vi "Mysql data reader Scalar double.vi"(8 "error in (no error)":errorcluster, 11 ".NET Refnum in":refnum<k24>) -> (0 "error out":errorcluster, 3 "GetString":dbl)   [LabVIEW 2020, in "mysql.lvlib" / "mysql.lvclass"]
uses:
  mysql.lvclass
  MySql.Data
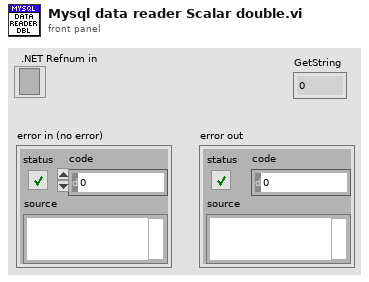
[diagram p1: front panel]
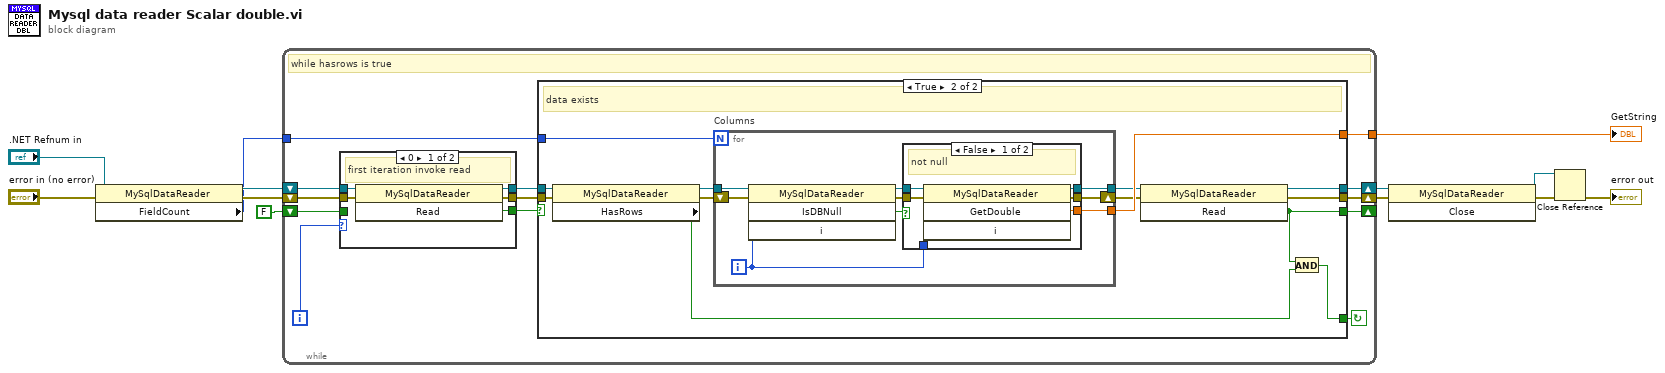
[diagram p0: block diagram]
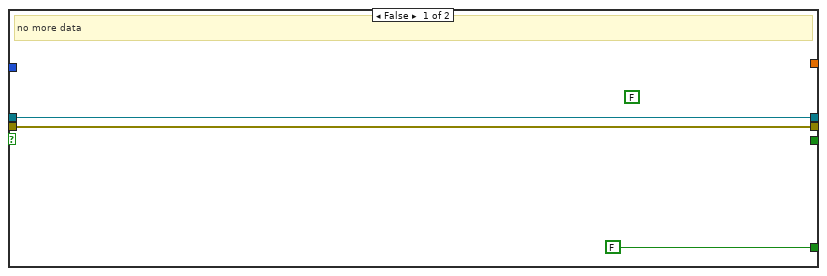
[diagram p3: hidden frame]
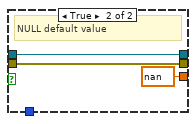
[diagram p4: hidden frame]
diagram:
  n1 = property class="MySqlDataReader"(reference=".NET Refnum in", error in="error in (no error)") -> (reference out=w8:refnum<k24>, error out=w7:errorcluster, "FieldCount"=w4:i32)
  n2 = while {
    tunnel: w4 -> [w25]
    tunnel: [w24] -> w5
    shift-right: [w22] -> w10
    shift-left: w7 -> [w20]
    shift-right: [w23] -> w9
    shift-left: w8 -> [w19]
    shift-right: [w13] -> _
    shift-left: FALSE -> [w15]
    i -> [w14]
    stop <- w21 continue-if-true
    # "while hasrows is true"
    n3 = case shown="0" w14 {
      tunnel: w20 -> [w30 w32]
      tunnel: [w29 w32] -> w17
      tunnel: w19 -> [w28 w33]
      tunnel: [w27 w33] -> w18
      tunnel: [w26 w31] -> w16
      tunnel: w15 -> [_ w31]
      frame 0 {
        # "first iteration invoke read"
        n4 = invoke class="MySqlDataReader" method="Read"(reference=w28, error in=w30) -> (reference out=w27:refnum<k24>, error out=w29:errorcluster, "Read"=w26:bool)  [unwired: 1 in]
      }
      frame 1.., Default {
        # "read after for other iterations"
      }
    }
    n5 = case shown="True" w16 {
      tunnel: w25 -> [_ w49]
      tunnel: [_ w48] -> w24
      tunnel: w17 -> [w35 w47]
      tunnel: w18 -> [w36 w46]
      tunnel: [w36 w43] -> w23
      tunnel: [w35 w41] -> w22
      tunnel: [FALSE ("HasRows") w38] -> w21
      tunnel: [_ w37] -> w13
      frame False {
        (unwired) FALSE
        # "no more data"
      }
      frame True {
        # "data exists"
        n6 = property class="MySqlDataReader"(reference=w46, error in=w47) -> (reference out=w45:refnum<k24>, error out=w44:errorcluster, "HasRows"=w39:bool)
        n7 = for "Columns" {
          N: w49 -> [_]
          tunnel: w45 -> [w53]
          shift-right: [w58] -> w42
          shift-left: w44 -> [w54]
          tunnel: [w57] -> w48
          tunnel: [w56] -> w40
          i -> [w55]
          n8 = invoke class="MySqlDataReader" method="IsDBNull"(reference=w53, error in=w54, "i"=w55) -> (reference out=w52:refnum<k24>, error out=w51:errorcluster, "IsDBNull"=w50:bool)  [unwired: 1 in, 1 out]
          n9 = case shown="False" w50 {
            tunnel: [w64 w66] -> w58
            tunnel: [w63 nan ("GetDouble")] -> w57
            tunnel: [w62 w67] -> w56
            tunnel: w55 -> [w61 _]
            tunnel: w52 -> [w60 w67]
            tunnel: w51 -> [w59 w66]
            frame False {
              # "not null"
              n10 = invoke class="MySqlDataReader" method="GetDouble"(reference=w60, error in=w59, "i"=w61) -> (reference out=w62:refnum<k24>, error out=w64:errorcluster, "GetDouble"=w63:dbl)  [unwired: 1 in, 1 out]
            }
            frame True {
              # "NULL default value"
            }
          }
        }
        n11 = invoke class="MySqlDataReader" method="Read"(reference=w40, error in=w42) -> (reference out=w43:refnum<k24>, error out=w41:errorcluster, "Read"=w37:bool)  [unwired: 1 in]
        n12 = And(x=w37, y=w39) -> (x .and. y?=w38:bool)
      }
    }
  }
  "GetString" <- w5
  n13 = invoke class="MySqlDataReader" method="Close"(reference=w9, error in=w10) -> (reference out=w12:refnum<k24>, error out=w11:errorcluster)  [unwired: 1 in, 1 out]
  n14 = Close Reference(reference=w12, error in (no error)=w11) -> (error out=→"error out":errorcluster)
